vi "Read Floor Selection.vi"(8 "error in (no error)":errorcluster, 11 "User Console in":refnum<class "User Console.lvclass">) -> (0 "error out":errorcluster, 2 "Floor Selection":T1, 3 "User Console out":refnum<class "User Console.lvclass">)   [LabVIEW 2019, in "User Console Actor.lvlib" / "User Console.lvclass"]
uses:
  User Console.lvclass
  Floor Selection.ctl
  User Console.lvclass/User Console.ctl
  Abstract User Console Actor/Abstract User Console Actor/Abstract User Console.lvclass
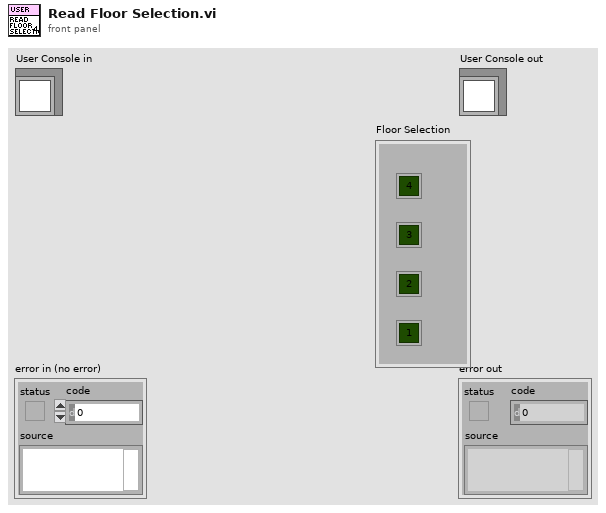
[diagram p1: front panel]
types:
  T1 = typedef "User Console Actor.lvlib/User Console.lvclass/Floor Selection.ctl" = cluster{"Floor4":bool, "Floor 3":bool, "Floor2":bool, "Floor1":bool}
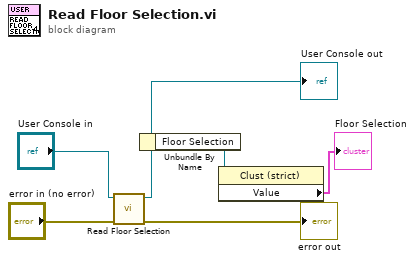
[diagram p0: block diagram]
diagram:
  n1 = call-parent "Read Floor Selection.vi"("error in (no error)"="error in (no error)", "Abstract User Console in"="User Console in") -> ("error out"=→"error out":errorcluster, "Abstract User Console out"=w3:refnum<class "User Console.lvclass">)  [unwired: 7 in, 1 out]
  "User Console out" <- w3
  n2 = Unbundle By Name(w3) -> ("Floor Selection"=w2:refnum<vi>)
  n3 = property class="Clust (strict)"(reference=w2) -> ("Value"=→"Floor Selection":T1)  [unwired: 1 in, 2 out]
